vi "Build Data Frame (Std 2011).vi"(8 "error in (no error)":errorcluster, 9 "system info in":refnum<class "PMU System Info.lvclass">, 11 "measurement data":T1 {"data error" format="%02b"; "PMU time quality" format="%03b"; "time quality flag" format="%08b"; "trigger reason" format="%04b"}) -> (0 "error out":errorcluster, 1 "system info out":refnum<class "PMU System Info.lvclass">, 3 "data frame":string)   [LabVIEW 2014, in "NI_EP_PMU.lvlib"]
doc: "Builds a data frame as defined in IEEE Std C37.118.2-2011."
uses:
  <vilib>/addons/Electrical Power/PMU/NI_EP_PMU.lvlib
  <vilib>/addons/Electrical Power/PMU/Common/Classes/PMU System Info/PMU System Info.lvclass
  <vilib>/addons/Electrical Power/PMU/Common/Controls/pmu_Measurement Data (Std 2011).ctl
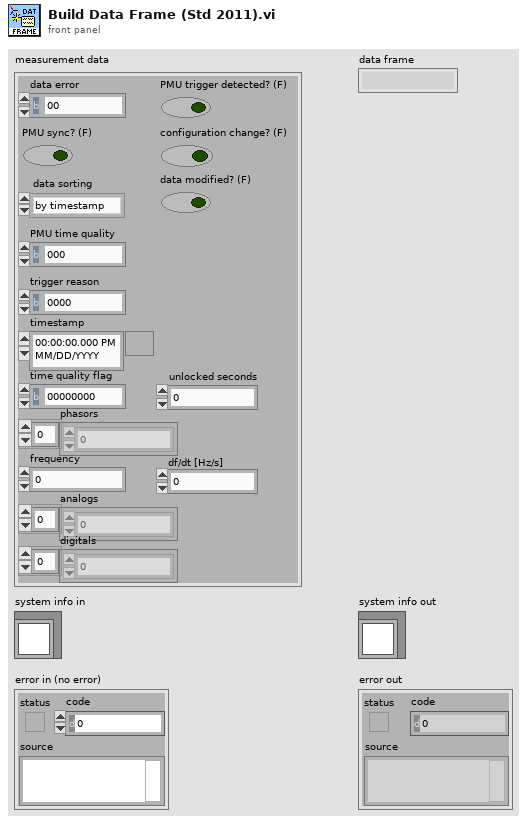
[diagram p1: front panel]
types:
  T1 = typedef "NI_EP_PMU.lvlib/pmu_Measurement Data (Std 2011).ctl" = cluster{"data error":u8, "PMU sync? (F)":bool, "data sorting":enum16{"by timestamp", "by arrival"}, "PMU trigger detected? (F)":bool, "configuration change? (F)":bool, "data modified? (F)":bool, "PMU time quality":u8, "trigger reason":u8, "timestamp":timestamp, "time quality flag":u8, "unlocked seconds":u32, "phasors":csg[], "frequency":sgl, "df/dt [Hz/s]":sgl, "analogs":sgl[], "digitals":u16[]}
  T2 = typedef "NI_EP_PMU.lvlib/pmu_CFG for Data Frame.ctl" = enum8{"CFG-2", "CFG-3"}
  T3 = typedef "NI_EP_PMU.lvlib/pmu_CFG Class.ctl" = cluster{"station name":string, "PMU ID":u16, "time base":u32, "nominal frequency":enum16{"50 Hz", "60 Hz"}, "reporting rate":i16, "phasor number":u16, "analog number":u16, "digital number":u16, "channel names":string[], "phasor units":u32[], "analog units":u32[], "digital units":u32[], "data format":u16, "number of PMUs":u16}
  T4 = typedef "NI_EP_PMU.lvlib/pmu_CFG-3 Class.ctl" = cluster{"station name":string, "PMU ID":u16, "global PMU ID":u64, "time base":u32, "nominal frequency":enum16{"50 Hz", "60 Hz"}, "reporting rate":i16, "phasor number":u16, "analog number":u16, "digital number":u16, "channel names":string[], "phasor scale first 4 bytes":u32[], "phasor scale factors":sgl[], "phasor angle offsets [rad]":sgl[], "analog scale factors":sgl[], "analog magnitude offsets":sgl[], "digital units":u32[], "data format":u16, "number of PMUs":u16}
  T5 = typedef "LVDateTimeRec.ctl" = cluster{"fractional second":dbl, "second":i32, "minute":i32, "hour":i32, "day of month":i32, "month":i32, "year":i32, "day of week":i32, "day of year":i32, "DST":i32}
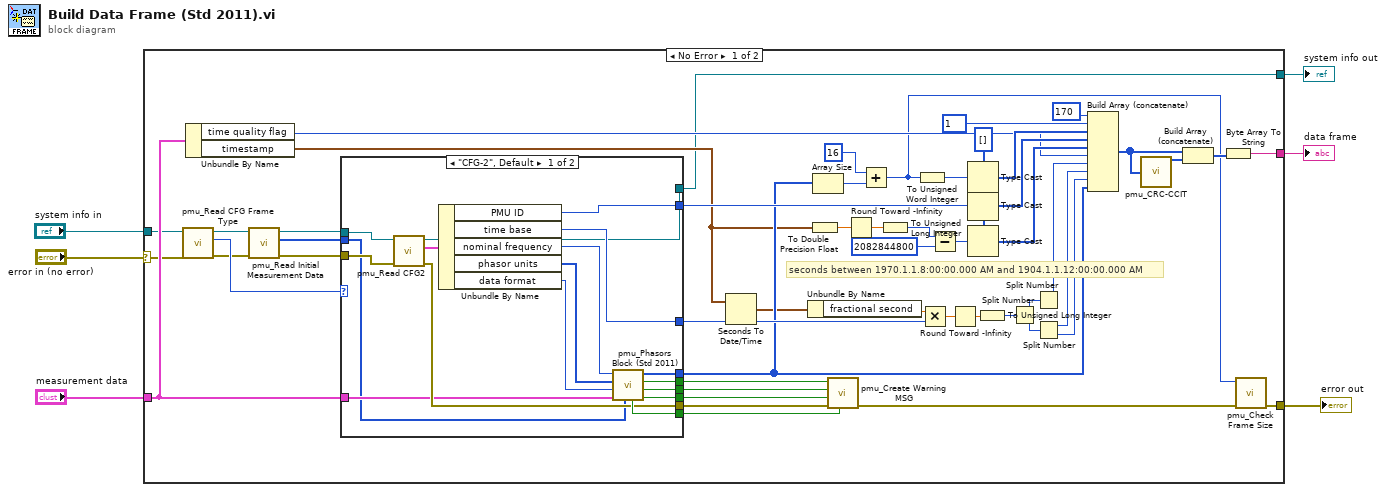
[diagram p0: block diagram]
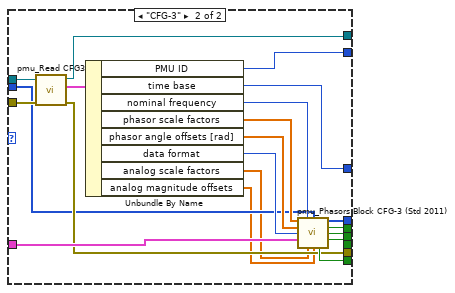
[diagram p2: hidden frame]
diagram:
  n1 = case shown="No Error" "error in (no error)" {
    selector: "error in (no error)" -> [w20 w95]
    tunnel: [w57 _] -> w6
    tunnel: "system info in" -> [w21 w96]
    tunnel: "measurement data" -> [w25 _]
    tunnel: [w10 w96] -> w3
    tunnel: [w11 w95] -> w2
    frame No Error {
      w53 = u8[] [] ("appended array")
      # "seconds between 1970.1.1.8:00:00.000 AM and 1904.1.1.12:00:00.000 AM"
      n2 = call <vilib>:"pmu_Read CFG Frame Type.vi"("error in (no error)"=w20, "system info in"=w21) -> ("error out"=w17:errorcluster, "configuration frame option"=w19:T2, "system info out"=w18:refnum<class "PMU System Info.lvclass">)  [unwired: 7 in]
      n3 = Unbundle By Name(w25) -> ("time quality flag"=w24:u8, "timestamp"=w22:timestamp)
      n4 = call <vilib>:"pmu_Read Initial Measurement Data.vi"("error in (no error)"=w17, "system info in"=w18) -> ("error out"=w14:errorcluster, "init meas data"=w16:u8[], "system info out"=w15:refnum<class "PMU System Info.lvclass">)  [unwired: 7 in]
      n5 = case shown="\"CFG-2\", Default" w19 {
        tunnel: [w73 w85] -> w38
        tunnel: [w72 w84] -> w37
        tunnel: [w70 w90] -> w36
        tunnel: [w69 w91] -> w10
        tunnel: w16 -> [w58 w77]
        tunnel: [w67 w89] -> w30
        tunnel: [w66 w88] -> w29
        tunnel: [w65 w87] -> w28
        tunnel: [w64 w86] -> w27
        tunnel: [w63 w78] -> w26
        tunnel: w25 -> [w62 w83]
        tunnel: w15 -> [w61 w94]
        tunnel: w14 -> [w60 w93]
        frame "CFG-2", Default {
          n6 = call <vilib>:"pmu_Read CFG2.vi"("error in (no error)"=w60, "system info in"=w61) -> ("error out"=w63:errorcluster, "CFG-2"=w74:T3, "system info out"=w69:refnum<class "PMU System Info.lvclass">)  [unwired: 7 in]
          n7 = Unbundle By Name(w74) -> ("PMU ID"=w72:u16, "time base"=w73:u32, "nominal frequency"=w59:enum16{"50 Hz", "60 Hz"}, "phasor units"=w71:u32[], "data format"=w68:u16)
          n8 = call <vilib>:"pmu_Phasors Block (Std 2011).vi"("init meas data"=w58, "measurement data"=w62, "data format"=w68, "phasor units"=w71, "nominal frequency"=w59) -> ("df/dt out of range"=w65:bool, "freq out of range"=w66:bool, "phasor out of range"=w67:bool, "data block"=w70:u8[], "analog out of range"=w64:bool)  [unwired: 2 in]
        }
        frame "CFG-3" {
          n9 = call <vilib>:"pmu_Read CFG3.vi"("error in (no error)"=w93, "system info in"=w94) -> ("error out"=w78:errorcluster, "CFG-3"=w92:T4, "system info out"=w91:refnum<class "PMU System Info.lvclass">)  [unwired: 7 in]
          n10 = Unbundle By Name(w92) -> ("PMU ID"=w84:u16, "time base"=w85:u32, "nominal frequency"=w79:enum16{"50 Hz", "60 Hz"}, "phasor scale factors"=w80:sgl[], "phasor angle offsets [rad]"=w81:sgl[], "data format"=w82:u16, "analog scale factors"=w76:sgl[], "analog magnitude offsets"=w75:sgl[])
          n11 = call <vilib>:"pmu_Phasors Block CFG-3 (Std 2011).vi"("phasor scale factors"=w80, "nominal frequency"=w79, "init meas data"=w77, "phasor angle offsets [rad]"=w81, "data format"=w82, "measurement data"=w83, "analog scale factors"=w76, "analog magnitude offsets"=w75) -> ("data block"=w90:u8[], "phasor out of range"=w89:bool, "freq out of range"=w88:bool, "df/dt out of range"=w87:bool, "analog out of range"=w86:bool)  [unwired: 3 in]
        }
      }
      n12 = Seconds To Date/Time(time stamp (now)=w22) -> (date time rec=w23:T5)  [unwired: 1 in]
      n13 = Unbundle By Name(w23) -> ("fractional second"=w56:dbl)
      n14 = To Double Precision Float(number=w22) -> (double precision float=w34:dbl)
      n15 = Array Size(array=w36) -> (size(s)=w9:i32)
      n16 = call <vilib>:"pmu_Create Warning MSG.vi"("analog out of range"=w27, "error in (no error)"=w26, "df/dt out of range"=w28, "freq out of range"=w29, "phasor out of range"=w30) -> ("error out"=w13:errorcluster)  [unwired: 6 in]
      n17 = Round Toward -Infinity(1:w34) -> (0:w33:dbl)
      n18 = Add(x=16 ("y"), y=w9) -> (x+y=w7:i32)
      n19 = To Unsigned Long Integer(number=w33) -> (unsigned 32bit integer=w55:u32)
      n20 = To Unsigned Word Integer(number=w7) -> (unsigned 16bit integer=w8:u16)
      n21 = Multiply(x=w56, y=w38) -> (x*y=w31:dbl)
      n22 = Subtract(x=w55, y=u32 2082844800 ("unsigned 32bit integer")) -> (x-y=w51:u32)
      n23 = Round Toward -Infinity(1:w31) -> (0:w32:dbl)
      n24 = Type Cast(type=w53, x=w8) -> (*(type *) &x=w49:u8[])
      n25 = Type Cast(type=w53, x=w37) -> (*(type *) &x=w50:u8[])
      n26 = Type Cast(type=w53, x=w51) -> (*(type *) &x=w52:u8[])
      n27 = To Unsigned Long Integer(number=w32) -> (unsigned 32bit integer=w54:u32)
      n28 = Split Number(x=w54) -> (hi(x)=w43:u16, lo(x)=w42:u16)
      n29 = Split Number(x=w43) -> (lo(x)=w44:u8)  [unwired: 1 out]
      n30 = Split Number(x=w42) -> (hi(x)=w45:u8, lo(x)=w46:u8)
      n31 = Build Array (concatenate)(u8 170 ("element"), u8 1 ("element"), w49, w50, w52, w24, w44, w45, w46, w36) -> (w47:u8[])
      n32 = call <vilib>:"pmu_CRC-CCIT.vi"("byte array"=w47) -> ("CRCbytes"=w48:u8[])  [unwired: 13 in, 1 out]
      n33 = Build Array (concatenate)(w47, w48) -> (w12:u8[])
      n34 = Byte Array To String(unsigned byte array=w12) -> (string=w57:string)
      n35 = call <vilib>:"pmu_Check Frame Size.vi"("error in (no error)"=w13, "frame size"=w7) -> ("error out"=w11:errorcluster)  [unwired: 9 in]
    }
    frame Error {
    }
  }
  "data frame" <- w6
  "error out" <- w2
  "system info out" <- w3
